vi "API_DB.UpdateLocationStatus.vi"(0 "Database in":refnum<class "Database.lvclass">, 1 "Wait (F)":bool, 2 "InventoryRecord.Location.Module":u16, 3 "InventoryRecord.LocationStatus":T1, 5 "Table":string, 7 "InventoryRecord.Stocker":T2 items=["Main", "Exp1", "Exp2"], 11 "error in (no error)":errorcluster, 12 "Timeout (ms)":u32, 13 "InventoryRecord.Location.Row":u16, 14 "InventoryRecord.Location.Column":u16) -> (4 "Database out":refnum<class "Database.lvclass">, 6 "Slot":string, 15 "error out":errorcluster)   [LabVIEW 2020, in "Database.lvclass"]
doc: "Developed by Kevin Thompson\nkevin@thompsonengineering.net\n\nCopyright 2018\nThompson Engineering, LLC"
uses:
  Database.lvclass
  DataTypes/Stocker--Enum.ctl
  DataTypes/LocationStatus--Enum.ctl
  DataTypes/AsynCmd_Temp01--enum.ctl
  DataTypes/GenericQuery--Cluster.ctl
  DataTypes/SQLQuery--Enum.ctl
  DataTypes/InventoryRecord--Cluster.ctl
  DataTypes/Module--Cluster.ctl
  Database.lvclass/Database.ctl
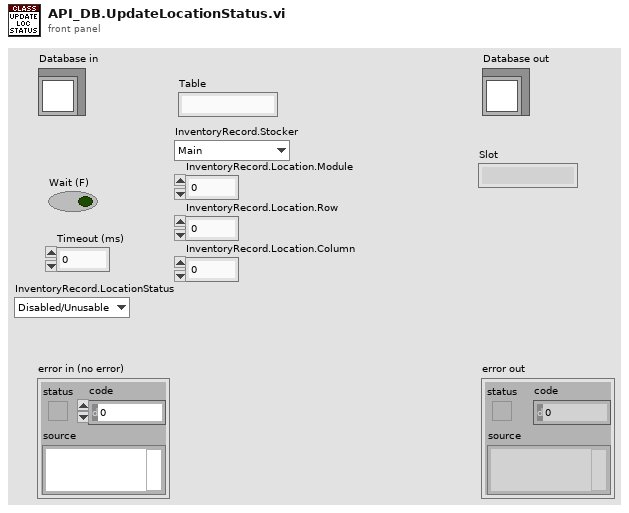
[diagram p1: front panel]
types:
  T1 = typedef "LocationStatus--Enum.ctl" = enum16{"Disabled/Unusable", "Full", "Empty"}
  T2 = typedef "Stocker--Enum.ctl" = u16
  T3 = typedef "SQLQuery--Enum.ctl" = enum16{"GetInventoryRecordFromDB", "GetReticleInfoFromDB", "GetLocationStatusFromDB", "UpdateInventoryRecord", "UpdateLocationStatus", "UpdateReticleLocationStatus", "AddReticleInDB", "RemoveReticleAtLocation", "RemoveReticleUsingReticleID", "GetLocationForReticleID", "GetAllLocations", "GetAllEmptyLocations", "GetAllLocationsInStocker", "GetAllFullLocations", "GetAllFullLocationsInStocker", "GetAllDisabledLocations", "GetAllDisabledLocationsInStocker", "FindFirstSlot"}
  T4 = typedef "GenericQuery--Cluster.ctl" = cluster{"Query":T3, "Table":string, "InventoryRecord":T5}
  T5 = typedef "InventoryRecord--Cluster.ctl" = cluster{"ReticleID":string, "Stocker":T2, "Location":T6, "LocationStatus":T1, "EquipmentID":string, "LocationID":string}
  T6 = typedef "Module--Cluster.ctl" = cluster{"Module":u16, "Row":u16, "Column":u16}
  T7 = typedef "Database.lvclass/AsynCmd_Temp01--enum.ctl" = enum16{"DB.DeleteRecord", "DB.UpdateRecord", "DB.InsertRecord", "DB.SelectRecord", "DB.ExecuteSQLCommand", "DB.FindFirstSlot", "DB.GenericSQLQuery"}
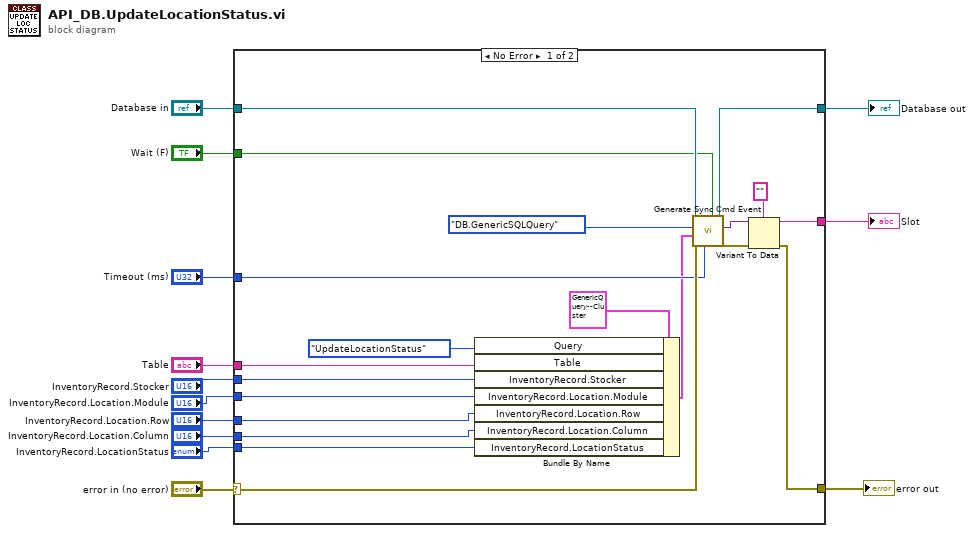
[diagram p0: block diagram]
diagram:
  n1 = case shown="No Error" "error in (no error)" {
    selector: "error in (no error)" -> [w31 w35]
    tunnel: [w26 w35] -> w12
    tunnel: [w32 w34] -> w10
    tunnel: "Database in" -> [w33 w34]
    tunnel: [w28 _] -> w7
    tunnel: "Wait (F)" -> [w25 _]
    tunnel: "Timeout (ms)" -> [w24 _]
    tunnel: "Table" -> [w19 _]
    tunnel: "InventoryRecord.Stocker" -> [w18 _]
    tunnel: "InventoryRecord.Location.Module" -> [w17 _]
    tunnel: "InventoryRecord.Location.Row" -> [w16 _]
    tunnel: "InventoryRecord.Location.Column" -> [w15 _]
    tunnel: "InventoryRecord.LocationStatus" -> [w14 _]
    frame No Error {
      n2 = Bundle By Name(cluster=T4 {"Query"=enum."GetInventoryRecordFromDB", "Table"="", "InventoryRecord"={"ReticleID"="", "Stocker"=0, "Location"={"Module"=0, "Row"=0, "Column"=0}, "LocationStatus"=enum."Disabled/Unusable", "EquipmentID"="", "LocationID"=""}}, "Query"=SQLQuery--Enum."UpdateLocationStatus", "Table"=w19, "InventoryRecord.Stocker"=w18, "InventoryRecord.Location.Module"=w17, "InventoryRecord.Location.Row"=w16, "InventoryRecord.Location.Column"=w15, "InventoryRecord.LocationStatus"=w14) -> (w20:T4)
      n3 = call "Generate Sync Cmd Event.vi"("Wait (F)"=w25, "Timeout (ms)"=w24, "error in (no error)"=w31, "vData"=w20, "AsyncCmd"=AsynCmd_Temp01--enum."DB.GenericSQLQuery", "Database in"=w33) -> ("error out"=w27:errorcluster, "Return Value"=w29:variant, "Database out"=w32:refnum<class "Database.lvclass">)  [unwired: 3 in]
      n4 = Variant To Data(error in=w27, type="", Variant=w29) -> (data=w28:string, error out=w26:errorcluster)
    }
    frame Error {
    }
  }
  "error out" <- w12
  "Database out" <- w10
  "Slot" <- w7
